vi "Run.vi"(8 "error in (no error)":errorcluster, 11 "Channel in":refnum<class "Channel.lvclass">) -> (0 "error out":errorcluster, 3 "Channel out":refnum<class "Channel.lvclass">)   [LabVIEW 2018, in "Channel.lvclass"]
uses:
  Channel.lvclass
  State Machine/State Machine.lvclass/State Machine.ctl
  Channel.lvclass/Channel.ctl
  State Machine/State Machine.lvclass
  RxTx/RxTx.lvclass
  Interface/Interface.lvclass
  TCS/TCS.lvclass
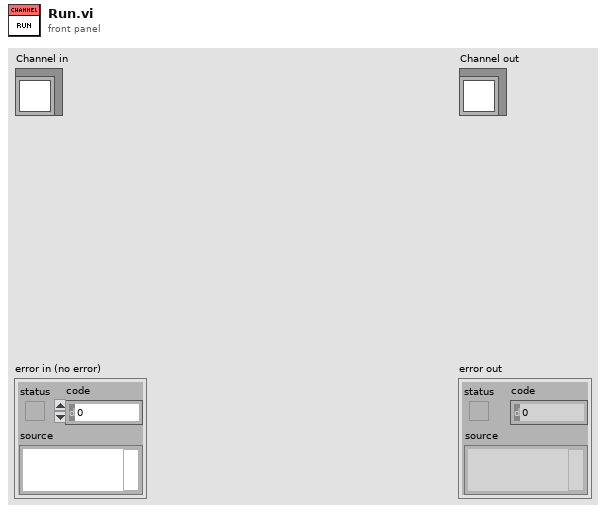
[diagram p1: front panel]
types:
  T1 = typedef "Shutter_mode typedef.ctl" = enum16{"Auto", "Open", "Close", "N/A (3)", "Open FVB Series", "Open Any Series"}
  T2 = typedef "ReadMode_mode typedef.ctl" = enum16{"Full Vertical Binning", "Multi-Track", "Random-Track", "Single-Track", "Image"}
  T3 = typedef "AcquisitionMode_mode typedef.ctl" = enum16{"Reserved (0)", "Single Scan", "Accumulate", "Kinetics", "Fast Kinetics", "Run Till Abort", "Reserved (6)", "Reserved (7)", "Reserved (8)", "Time Delayed Integration"}
  T4 = cluster{"EXPTIME":sgl, "PREAMP":enum16{"Gain 1", "Gain 2"}, "READOUT_RATE":enum16{"30 MHz", "20 MHz", "10 MHz", "1 MHz"}, "EM_GAIN":u16, "VBIN":u16, "INITIAL_LINE":u16, "INITIAL_COLUMN":u16, "FINAL_LINE":u16, "FINAL_COLUMN":u16, "#FRAMES":u32, "#CUBES":u32, "TRIGGER_MODE":enum16{"Internal", "External", "N/A", "N/A_1", "N/A_2", "N/A_3", "External Start"}, "HBIN":u16, "SHUTTER_TTL":enum16{"TTL Low", "TTL High"}, "SHUTTER_MODE":T1, "SHUTTER_OPENING_TIME":u16, "SHUTTER_CLOSING_TIME":u16, "VERTICAL_SHIFT_SPEED":u16, "READ_MODE":T2, "FRAME_TRANSFER":bool, "VERTICAL_CLOCK_VOLTAGE":enum16{"0", "+1", "+2", "+3", "+4"}, "ACQUISITION_MODE":T3, "AD_CHANNEL":u16, "EM_MODE":enum16{"Electron Multiplying", "Conventional"}}
  T5 = cluster{"CUBE_EXPOSURE_TIME":sgl, "CUBES_DONE":u16, "LAST_IMAGE_NAME":string, "DISK_SPACE":u16, "FRAMES_DONE":u16, "CCD_STATUS":string, "CURRENT_TEMPERATURE":i16, "TEMPERATURE_STATUS":string, "FRAME_EXPOSURE_TIME":u16, "CCD_ON_OFF":bool, "SERIAL_NUMBER":u16, "ACQUIRING":bool}
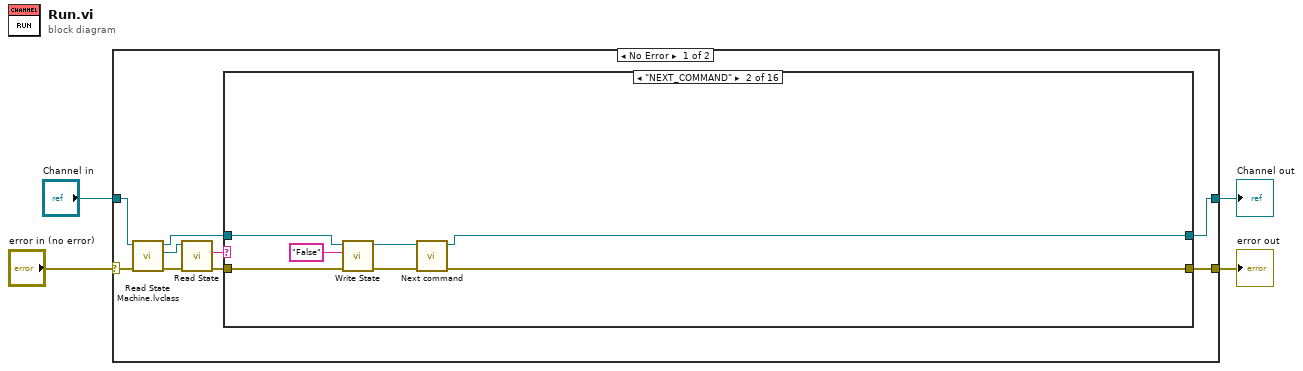
[diagram p0: block diagram]
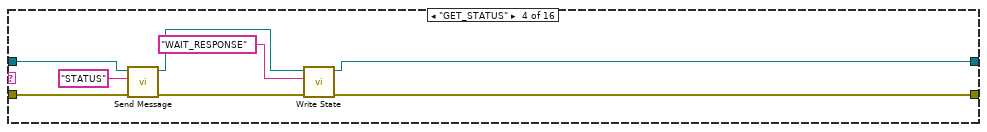
[diagram p4: hidden frame]
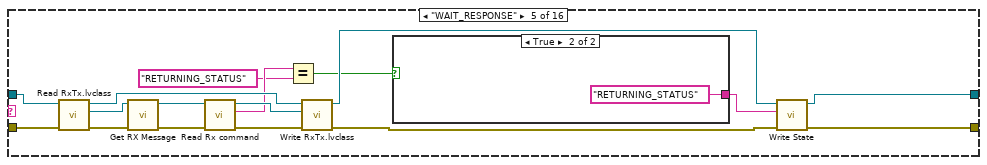
[diagram p5: hidden frame]
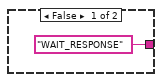
[diagram p6: hidden frame]
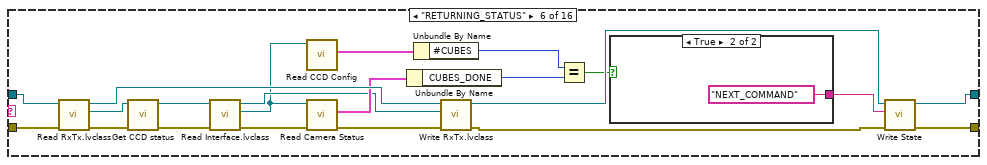
[diagram p7: hidden frame]
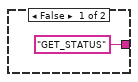
[diagram p8: hidden frame]
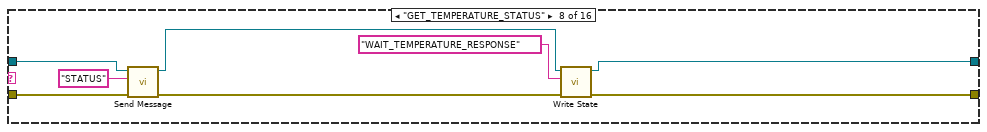
[diagram p10: hidden frame]
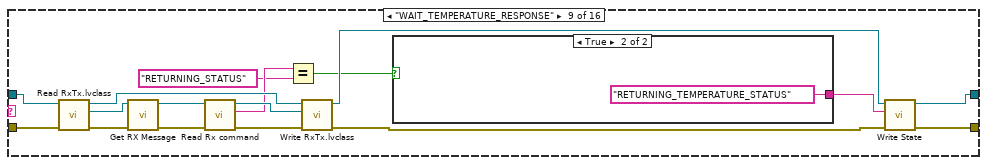
[diagram p11: hidden frame]
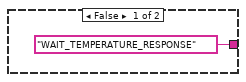
[diagram p12: hidden frame]
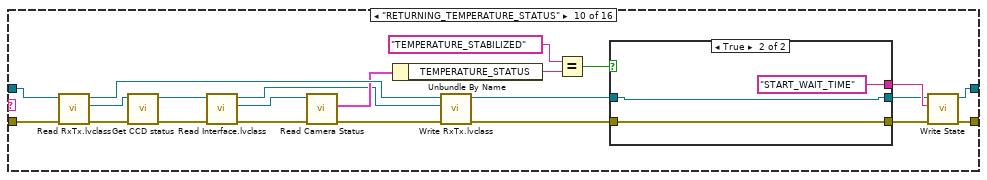
[diagram p13: hidden frame]
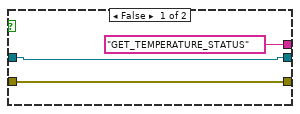
[diagram p14: hidden frame]
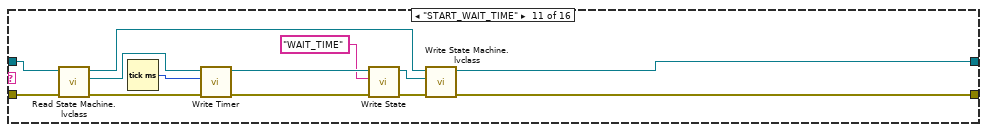
[diagram p15: hidden frame]
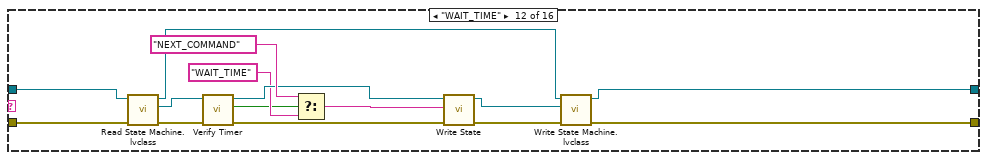
[diagram p16: hidden frame]
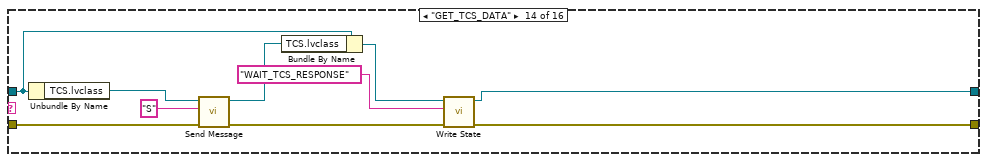
[diagram p18: hidden frame]
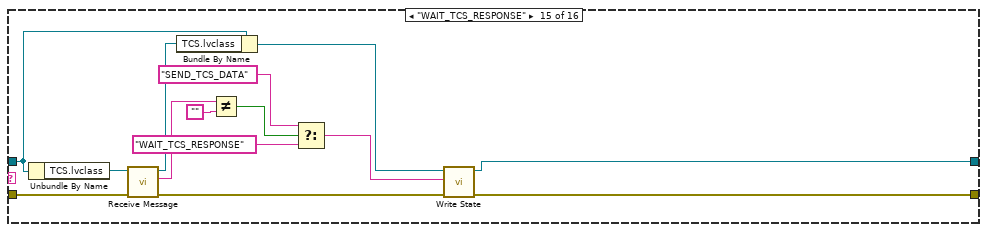
[diagram p19: hidden frame]
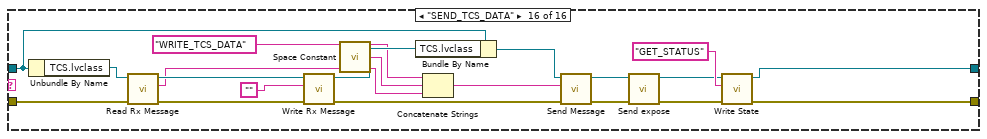
[diagram p20: hidden frame]
diagram:
  n1 = case shown="No Error" "error in (no error)" {
    selector: "error in (no error)" -> [w8 w207]
    tunnel: [w5 w207] -> w3
    tunnel: [w6 w206] -> w1
    tunnel: "Channel in" -> [w7 w206]
    frame No Error {
      n2 = call "Read State Machine.lvclass.vi"("error in (no error)"=w8, "Channel in"=w7) -> ("error out"=w12:errorcluster, "State Machine.lvclass"=w13:refnum<class "State Machine.lvclass">, "Channel out"=w10:refnum<class "Channel.lvclass">)  [unwired: 7 in]
      n3 = call-dynamic "Read State.vi"("error in (no error)"=w12, "State Machine in"=w13) -> ("error out"=w9:errorcluster, "State"=w11:string)  [unwired: 7 in, 1 out]
      n4 = case shown="\"NEXT_COMMAND\"" w11 {
        tunnel: w10 -> [w15 w21 w23 w32 w49 w72 w76 w84 w88 w125 w144 w159 w161 w168 w185 w205]
        tunnel: w9 -> [w14 w22 w24 w31 w48 w71 w75 w83 w89 w124 w143 w158 w160 w170 w178 w197]
        tunnel: [w15 w19 w23 w27 w37 w68 w76 w79 w87 w121 w135 w155 w161 w165 w183 w204] -> w6
        tunnel: [w14 w18 w24 w26 w38 w69 w75 w78 w86 w122 w136 w156 w160 w164 w182 w203] -> w5
        frame "False", Default {
        }
        frame "NEXT_COMMAND" {
          n5 = call "Write State.vi"("error in (no error)"=w22, "State"="False", "Channel in"=w21) -> ("error out"=w17:errorcluster, "Channel out"=w20:refnum<class "Channel.lvclass">)  [unwired: 7 in]
          n6 = call "Next command.vi"("error in (no error)"=w17, "Channel in"=w20) -> ("error out"=w18:errorcluster, "Channel out"=w19:refnum<class "Channel.lvclass">)  [unwired: 8 in]
        }
        frame "N/A2" {
        }
        frame "GET_STATUS" {
          n7 = call "Send Message.vi"("error in (no error)"=w31, "message"="STATUS", "Channel in"=w32) -> ("error out"=w28:errorcluster, "Channel out"=w29:refnum<class "Channel.lvclass">)  [unwired: 7 in]
          n8 = call "Write State.vi"("error in (no error)"=w28, "State"="WAIT_RESPONSE" ("message"), "Channel in"=w29) -> ("error out"=w26:errorcluster, "Channel out"=w27:refnum<class "Channel.lvclass">)  [unwired: 7 in]
        }
        frame "WAIT_RESPONSE" {
          n9 = call "Read RxTx.lvclass.vi"("error in (no error)"=w48, "Channel in"=w49) -> ("error out"=w45:errorcluster, "RxTx.lvclass"=w44:refnum<class "RxTx.lvclass">, "Channel out"=w41:refnum<class "Channel.lvclass">)  [unwired: 7 in]
          n10 = call "Get RX Message.vi"("error in (no error)"=w45, "RxTx in"=w44) -> ("error out"=w46:errorcluster, "RxTx out"=w47:refnum<class "RxTx.lvclass">)  [unwired: 8 in]
          n11 = call "Read Rx command.vi"("error in (no error)"=w46, "RxTx in"=w47) -> ("error out"=w43:errorcluster, "Rx Command"=w34:string, "RxTx out"=w42:refnum<class "RxTx.lvclass">)  [unwired: 7 in]
          n12 = Equal?(x=w34, y="RETURNING_STATUS") -> (x = y?=w36:bool)
          n13 = call "Write RxTx.lvclass.vi"("error in (no error)"=w43, "RxTx.lvclass"=w42, "Channel in"=w41) -> ("error out"=w39:errorcluster, "Channel out"=w40:refnum<class "Channel.lvclass">)  [unwired: 7 in]
          n14 = case shown="True" w36 {
            tunnel: ["WAIT_RESPONSE" "RETURNING_STATUS"] -> w35
            frame False {
            }
            frame True {
            }
          }
          n15 = call "Write State.vi"("error in (no error)"=w39, "State"=w35, "Channel in"=w40) -> ("error out"=w38:errorcluster, "Channel out"=w37:refnum<class "Channel.lvclass">)  [unwired: 7 in]
        }
        frame "RETURNING_STATUS" {
          n16 = call "Read RxTx.lvclass.vi"("error in (no error)"=w71, "Channel in"=w72) -> ("error out"=w66:errorcluster, "RxTx.lvclass"=w67:refnum<class "RxTx.lvclass">, "Channel out"=w70:refnum<class "Channel.lvclass">)  [unwired: 7 in]
          n17 = call "Get CCD status.vi"("error in (no error)"=w66, "RxTx in"=w67) -> ("error out"=w52:errorcluster, "RxTx out"=w53:refnum<class "RxTx.lvclass">)  [unwired: 8 in]
          n18 = call "Read Interface.lvclass.vi"("error in (no error)"=w52, "RxTx in"=w53) -> ("error out"=w65:errorcluster, "Interface.lvclass"=w60:refnum<class "Interface.lvclass">, "RxTx out"=w61:refnum<class "RxTx.lvclass">)  [unwired: 7 in]
          n19 = call "Read CCD Config.vi"("Interface in"=w60) -> ("CCD Config"=w59:T4)  [unwired: 8 in, 2 out]
          n20 = call "Read Camera Status.vi"("error in (no error)"=w65, "Interface in"=w60) -> ("error out"=w62:errorcluster, "Camera Status"=w64:T5)  [unwired: 7 in, 1 out]
          n21 = Unbundle By Name(w64) -> ("CUBES_DONE"=w55:u16)
          n22 = Unbundle By Name(w59) -> ("#CUBES"=w56:u32)
          n23 = call "Write RxTx.lvclass.vi"("error in (no error)"=w62, "RxTx.lvclass"=w61, "Channel in"=w70) -> ("error out"=w57:errorcluster, "Channel out"=w58:refnum<class "Channel.lvclass">)  [unwired: 7 in]
          n24 = Equal?(x=w56, y=w55) -> (x = y?=w54:bool)
          n25 = case shown="True" w54 {
            tunnel: ["GET_STATUS" ("State") "NEXT_COMMAND" ("State")] -> w63
            frame False {
            }
            frame True {
            }
          }
          n26 = call "Write State.vi"("error in (no error)"=w57, "State"=w63, "Channel in"=w58) -> ("error out"=w69:errorcluster, "Channel out"=w68:refnum<class "Channel.lvclass">)  [unwired: 7 in]
        }
        frame "N/A" {
        }
        frame "GET_TEMPERATURE_STATUS" {
          n27 = call "Send Message.vi"("error in (no error)"=w83, "message"="STATUS", "Channel in"=w84) -> ("error out"=w80:errorcluster, "Channel out"=w81:refnum<class "Channel.lvclass">)  [unwired: 7 in]
          n28 = call "Write State.vi"("error in (no error)"=w80, "State"="WAIT_TEMPERATURE_RESPONSE" ("message"), "Channel in"=w81) -> ("error out"=w78:errorcluster, "Channel out"=w79:refnum<class "Channel.lvclass">)  [unwired: 7 in]
        }
        frame "WAIT_TEMPERATURE_RESPONSE" {
          n29 = call "Read RxTx.lvclass.vi"("error in (no error)"=w89, "Channel in"=w88) -> ("error out"=w99:errorcluster, "RxTx.lvclass"=w98:refnum<class "RxTx.lvclass">, "Channel out"=w95:refnum<class "Channel.lvclass">)  [unwired: 7 in]
          n30 = call "Get RX Message.vi"("error in (no error)"=w99, "RxTx in"=w98) -> ("error out"=w100:errorcluster, "RxTx out"=w101:refnum<class "RxTx.lvclass">)  [unwired: 8 in]
          n31 = call "Read Rx command.vi"("error in (no error)"=w100, "RxTx in"=w101) -> ("error out"=w97:errorcluster, "Rx Command"=w90:string, "RxTx out"=w96:refnum<class "RxTx.lvclass">)  [unwired: 7 in]
          n32 = Equal?(x=w90, y="RETURNING_STATUS") -> (x = y?=w92:bool)
          n33 = call "Write RxTx.lvclass.vi"("error in (no error)"=w97, "RxTx.lvclass"=w96, "Channel in"=w95) -> ("error out"=w93:errorcluster, "Channel out"=w94:refnum<class "Channel.lvclass">)  [unwired: 7 in]
          n34 = case shown="True" w92 {
            tunnel: ["WAIT_TEMPERATURE_RESPONSE" "RETURNING_TEMPERATURE_STATUS"] -> w91
            frame False {
            }
            frame True {
            }
          }
          n35 = call "Write State.vi"("error in (no error)"=w93, "State"=w91, "Channel in"=w94) -> ("error out"=w86:errorcluster, "Channel out"=w87:refnum<class "Channel.lvclass">)  [unwired: 7 in]
        }
        frame "RETURNING_TEMPERATURE_STATUS" {
          n36 = call "Read RxTx.lvclass.vi"("error in (no error)"=w124, "Channel in"=w125) -> ("error out"=w119:errorcluster, "RxTx.lvclass"=w120:refnum<class "RxTx.lvclass">, "Channel out"=w123:refnum<class "Channel.lvclass">)  [unwired: 7 in]
          n37 = call "Get CCD status.vi"("error in (no error)"=w119, "RxTx in"=w120) -> ("error out"=w117:errorcluster, "RxTx out"=w118:refnum<class "RxTx.lvclass">)  [unwired: 8 in]
          n38 = call "Read Interface.lvclass.vi"("error in (no error)"=w117, "RxTx in"=w118) -> ("error out"=w115:errorcluster, "Interface.lvclass"=w116:refnum<class "Interface.lvclass">, "RxTx out"=w108:refnum<class "RxTx.lvclass">)  [unwired: 7 in]
          n39 = call "Read Camera Status.vi"("error in (no error)"=w115, "Interface in"=w116) -> ("error out"=w109:errorcluster, "Camera Status"=w114:T5)  [unwired: 7 in, 1 out]
          n40 = Unbundle By Name(w114) -> ("TEMPERATURE_STATUS"=w113:string)
          n41 = call "Write RxTx.lvclass.vi"("error in (no error)"=w109, "RxTx.lvclass"=w108, "Channel in"=w123) -> ("error out"=w107:errorcluster, "Channel out"=w105:refnum<class "Channel.lvclass">)  [unwired: 7 in]
          n42 = Equal?(x="TEMPERATURE_STABILIZED" ("State"), y=w113) -> (x = y?=w111:bool)
          n43 = case shown="True" w111 {
            tunnel: ["GET_TEMPERATURE_STATUS" ("State") "START_WAIT_TIME" ("State")] -> w110
            tunnel: w107 -> [w127 w129]
            tunnel: [w127 w129] -> w106
            tunnel: w105 -> [w126 w130]
            tunnel: [w126 w130] -> w104
            frame False {
            }
            frame True {
            }
          }
          n44 = call "Write State.vi"("error in (no error)"=w106, "State"=w110, "Channel in"=w104) -> ("error out"=w122:errorcluster, "Channel out"=w121:refnum<class "Channel.lvclass">)  [unwired: 7 in]
        }
        frame "START_WAIT_TIME" {
          n45 = call "Read State Machine.lvclass.vi"("error in (no error)"=w143, "Channel in"=w144) -> ("error out"=w141:errorcluster, "State Machine.lvclass"=w142:refnum<class "State Machine.lvclass">, "Channel out"=w137:refnum<class "Channel.lvclass">)  [unwired: 7 in]
          n46 = Tick Count (ms)() -> (millisecond timer value=w138:u32)
          n47 = call "Write Timer.vi"("error in (no error)"=w141, "Timer"=w138, "State Machine in"=w142) -> ("error out"=w139:errorcluster, "State Machine out"=w140:refnum<class "State Machine.lvclass">)  [unwired: 7 in]
          n48 = call-dynamic "Write State.vi"("error in (no error)"=w139, "State"="WAIT_TIME", "State Machine in"=w140) -> ("error out"=w133:errorcluster, "State Machine out"=w134:refnum<class "State Machine.lvclass">)  [unwired: 7 in]
          n49 = call "Write State Machine.lvclass.vi"("error in (no error)"=w133, "State Machine.lvclass"=w134, "Channel in"=w137) -> ("error out"=w136:errorcluster, "Channel out"=w135:refnum<class "Channel.lvclass">)  [unwired: 7 in]
        }
        frame "WAIT_TIME" {
          n50 = call "Read State Machine.lvclass.vi"("error in (no error)"=w158, "Channel in"=w159) -> ("error out"=w151:errorcluster, "State Machine.lvclass"=w152:refnum<class "State Machine.lvclass">, "Channel out"=w157:refnum<class "Channel.lvclass">)  [unwired: 7 in]
          n51 = call "Verify Timer.vi"("error in (no error)"=w151, "State Machine in"=w152) -> ("error out"=w147:errorcluster, "Time out"=w145:bool, "State Machine out"=w148:refnum<class "State Machine.lvclass">)  [unwired: 6 in, 1 out]
          n52 = Select(t="NEXT_COMMAND", s=w145, f="WAIT_TIME") -> (s? t:f=w149:string)
          n53 = call-dynamic "Write State.vi"("error in (no error)"=w147, "State"=w149, "State Machine in"=w148) -> ("error out"=w153:errorcluster, "State Machine out"=w154:refnum<class "State Machine.lvclass">)  [unwired: 7 in]
          n54 = call "Write State Machine.lvclass.vi"("error in (no error)"=w153, "State Machine.lvclass"=w154, "Channel in"=w157) -> ("error out"=w156:errorcluster, "Channel out"=w155:refnum<class "Channel.lvclass">)  [unwired: 7 in]
        }
        frame "N/A3" {
        }
        frame "GET_TCS_DATA" {
          n55 = Unbundle By Name(w168) -> ("TCS.lvclass"=w171:refnum<class "TCS.lvclass">)
          n56 = call "Send Message.vi"("error in (no error)"=w170, "message"="S", "TCS in"=w171) -> ("error out"=w163:errorcluster, "TCS out"=w167:refnum<class "TCS.lvclass">)  [unwired: 7 in]
          n57 = Bundle By Name(cluster=w168, "TCS.lvclass"=w167) -> (w166:refnum<class "Channel.lvclass">)
          n58 = call "Write State.vi"("error in (no error)"=w163, "State"="WAIT_TCS_RESPONSE", "Channel in"=w166) -> ("error out"=w164:errorcluster, "Channel out"=w165:refnum<class "Channel.lvclass">)  [unwired: 7 in]
        }
        frame "WAIT_TCS_RESPONSE" {
          n59 = Unbundle By Name(w185) -> ("TCS.lvclass"=w181:refnum<class "TCS.lvclass">)
          n60 = call "Receive Message.vi"("error in (no error)"=w178, "TCS in"=w181) -> ("error out"=w179:errorcluster, "Rx message"=w172:string, "TCS out"=w180:refnum<class "TCS.lvclass">)  [unwired: 7 in]
          n61 = Bundle By Name(cluster=w185, "TCS.lvclass"=w180) -> (w184:refnum<class "Channel.lvclass">)
          n62 = Not Equal?(x=w172, y="") -> (x != y?=w177:bool)
          n63 = Select(t="SEND_TCS_DATA" ("State"), s=w177, f="WAIT_TCS_RESPONSE" ("State")) -> (s? t:f=w173:string)
          n64 = call "Write State.vi"("error in (no error)"=w179, "State"=w173, "Channel in"=w184) -> ("error out"=w182:errorcluster, "Channel out"=w183:refnum<class "Channel.lvclass">)  [unwired: 7 in]
        }
        frame "SEND_TCS_DATA" {
          n65 = Unbundle By Name(w205) -> ("TCS.lvclass"=w202:refnum<class "TCS.lvclass">)
          n66 = call "Read Rx Message.vi"("error in (no error)"=w197, "TCS in"=w202) -> ("error out"=w199:errorcluster, "Rx message"=w194:string, "TCS out"=w201:refnum<class "TCS.lvclass">)  [unwired: 7 in]
          n67 = call "Write Rx Message.vi"("error in (no error)"=w199, "Rx message"="", "TCS in"=w201) -> ("error out"=w190:errorcluster, "TCS out"=w200:refnum<class "TCS.lvclass">)  [unwired: 7 in]
          n68 = call <vilib>:"Space Constant.vi"() -> ("String"=w195:string)
          n69 = Bundle By Name(cluster=w205, "TCS.lvclass"=w200) -> (w192:refnum<class "Channel.lvclass">)
          n70 = Concatenate Strings("WRITE_TCS_DATA", w195, w194) -> (w193:string)
          n71 = call "Send Message.vi"("error in (no error)"=w190, "message"=w193, "Channel in"=w192) -> ("error out"=w186:errorcluster, "Channel out"=w189:refnum<class "Channel.lvclass">)  [unwired: 7 in]
          n72 = call "Send expose.vi"("error in (no error)"=w186, "Channel in"=w189) -> ("error out"=w187:errorcluster, "Channel out"=w188:refnum<class "Channel.lvclass">)  [unwired: 8 in]
          n73 = call "Write State.vi"("error in (no error)"=w187, "State"="GET_STATUS", "Channel in"=w188) -> ("error out"=w203:errorcluster, "Channel out"=w204:refnum<class "Channel.lvclass">)  [unwired: 7 in]
        }
      }
    }
    frame Error {
    }
  }
  "error out" <- w3
  "Channel out" <- w1
